vi "LMS_SetLPFBW.vi"(6 "bandwidth":dbl, 8 "error in (no error)":errorcluster, 9 "chan":u64, 10 "dir_tx":u8, 11 "device_In":i64) -> (0 "error out":errorcluster, 3 "device_Out":i64)   [LabVIEW 2018, in "LMS_LV_Drv.lvlib"]
uses:
  LMS_LV_Drv.lvlib
  C:/Program Files/PothosSDR/bin/LimeSuite.dll
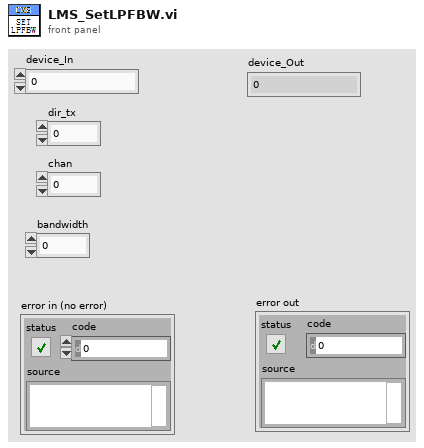
[diagram p1: front panel]
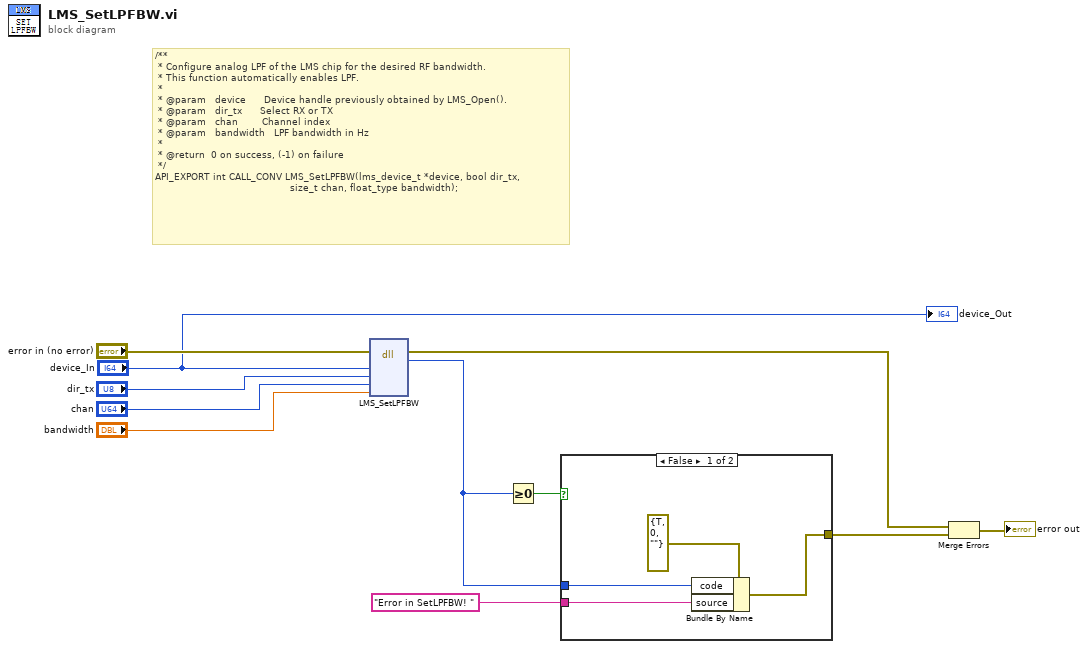
[diagram p0: block diagram]
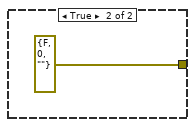
[diagram p2: hidden frame]
diagram:
  # "/**\n * Configure analog LPF of the LMS chip for the desired RF bandwidth.\n * This function automatically enables LPF.\n *\n * @param   device      Device handle previously obtained by LMS_Open().\n * @param   dir_tx      Select RX or TX\n * @param   chan        Channel index\n * @param   bandwidth   LPF bandwidth in Hz\n *\n * @return  0 on success, (-1) on failure\n */\nAPI_EXPORT int CALL_CONV LMS_SetLPFBW(lms_device_t *device, bool dir_tx,\n                                             size_t chan, float_type bandwidth);"
  n1 = dll-call lib="C:/Program Files/PothosSDR/bin/LimeSuite.dll" fn="LMS_SetLPFBW"(error in="error in (no error)", "device"="device_In", "dir_tx"="dir_tx", "chan"="chan", "bandwidth"="bandwidth") -> (error out=w2:errorcluster, "return type"=w3:i32)  [unwired: 6 in, 1 out]
  n2 = Greater Or Equal To 0?(x=w3) -> (x >= 0?=w6:bool)
  n3 = case shown="False" w6 {
    tunnel: [w14 errorcluster {"status"=FALSE, "code"=0, "source"=""} ("error in")] -> w4
    tunnel: w3 -> [w13 _]
    tunnel: "Error in SetLPFBW! " ("source") -> [w12 _]
    frame False {
      n4 = Bundle By Name(cluster=errorcluster {"status"=TRUE, "code"=0, "source"=""} ("error in"), "code"=w13, "source"=w12) -> (w14:errorcluster)
    }
    frame True {
    }
  }
  n5 = Merge Errors(w2, w4) -> (→"error out":errorcluster)
  "device_Out" <- "device_In"
